vi "Bai3_3_C1.vi"() -> ()   [LabVIEW 2019]
panel:
  in  "stop":bool
  out "Bit sang":i32
  in  "Stop":bool=TRUE
  in  "Lines to Write":u16(ring) items=["0 - 7", "8 - 15", "16 - 23"]
  in  "Device Name":tag="Dev8"
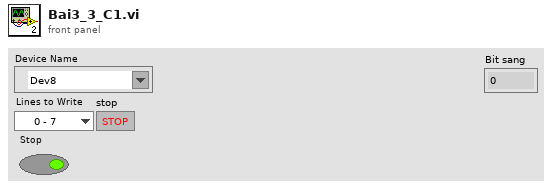
[diagram p1: front panel]
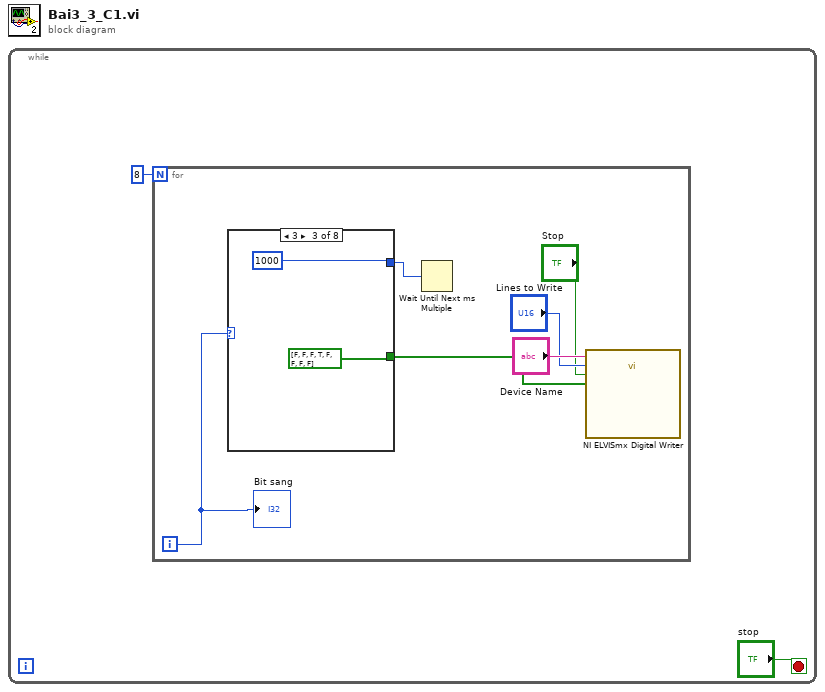
[diagram p0: block diagram]
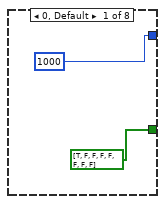
[diagram p2: hidden frame]
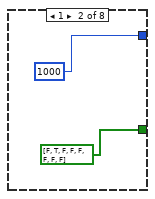
[diagram p3: hidden frame]
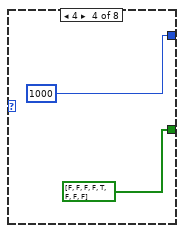
[diagram p4: hidden frame]
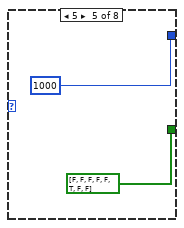
[diagram p5: hidden frame]
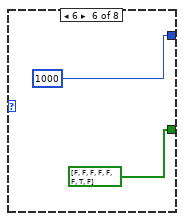
[diagram p6: hidden frame]
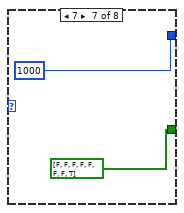
[diagram p7: hidden frame]
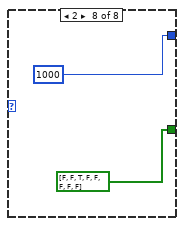
[diagram p8: hidden frame]
diagram:
  n1 = while {
    stop <- "stop" stop-if-true
    n2 = for {
      N: 8 -> [_]
      i -> [w5]
      n3 = case shown="3" w5 {
        tunnel: [u32 1000 ("millisecond multiple") u32 1000 ("millisecond multiple") u32 1000 ("millisecond multiple") u32 1000 ("millisecond multiple") u32 1000 ("millisecond multiple") u32 1000 ("millisecond multiple") u32 1000 ("millisecond multiple") u32 1000 ("millisecond multiple")] -> w4
        tunnel: [bool[] [TRUE, FALSE, FALSE, FALSE, FALSE, FALSE, FALSE, FALSE] ("DO Lines") bool[] [FALSE, TRUE, FALSE, FALSE, FALSE, FALSE, FALSE, FALSE] ("DO Lines") bool[] [FALSE, FALSE, FALSE, TRUE, FALSE, FALSE, FALSE, FALSE] ("DO Lines") bool[] [FALSE, FALSE, FALSE, FALSE, TRUE, FALSE, FALSE, FALSE] ("DO Lines") bool[] [FALSE, FALSE, FALSE, FALSE, FALSE, TRUE, FALSE, FALSE] ("DO Lines") bool[] [FALSE, FALSE, FALSE, FALSE, FALSE, FALSE, TRUE, FALSE] ("DO Lines") bool[] [FALSE, FALSE, FALSE, FALSE, FALSE, FALSE, FALSE, TRUE] ("DO Lines") bool[] [FALSE, FALSE, TRUE, FALSE, FALSE, FALSE, FALSE, FALSE] ("DO Lines")] -> w3
        frame 0, Default {
        }
        frame 1 {
        }
        frame 3 {
        }
        frame 4 {
        }
        frame 5 {
        }
        frame 6 {
        }
        frame 7 {
        }
        frame 2 {
        }
      }
      n4 = Wait Until Next ms Multiple(millisecond multiple=w4) -> ()  [unwired: 1 out]
      n5 = call "NI ELVISmx Digital Writer"("Device Name"="Device Name", "Lines to Write"="Lines to Write", "Stop"="Stop", "DO Lines"=w3) -> ()  [unwired: 15 in, 1 out]
      "Bit sang" <- w5
    }
  }
